vi "Initialize Core.vi"(8 "error in":errorcluster, 10 "Shared Resources":refnum<class "Shared Resources.lvclass">, 11 "Execution Unit in":refnum<class "Execution Unit.lvclass">) -> (0 "error out":errorcluster, 3 "Execution Unit out":refnum<class "Execution Unit.lvclass">)   [LabVIEW 2024, in "AIM ARINC 429 Engine.lvlib" / "Implementation.lvlib" / "Execution Unit.lvclass"]
uses:
  Execution Unit.lvclass
  Shared Resources/Shared Resources.lvclass
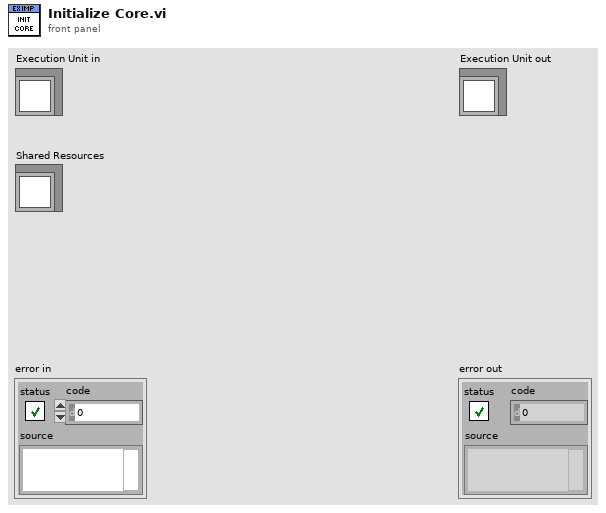
[diagram p1: front panel]
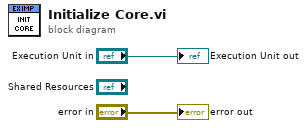
[diagram p0: block diagram]
diagram:
  "error out" <- "error in"
  "Execution Unit out" <- "Execution Unit in"
